vi "Get Altitude Data.vi"(8 "error in (no error)":errorcluster, 10 "Complete NMEA Sentences":string[](array[string]), 11 "VISA resource name":refnum<visa-resource-name>) -> (0 "error out":errorcluster, 1 "Altitude Data":cluster{"Timestamp":timestamp, "Altitude":dbl}[](array[cluster]), 2 "Complete NMEA Sentences (Copy)":string[](array[string]), 3 "VISA resource name out":refnum<visa-resource-name>)   [LabVIEW 2009]
doc: "Parses out the altitude data from all of the sentences that Read Raw.vi outputs, and passes through a complete copy of those sentences. Can be used in conjunction with other advanced \"Get\" VIs. See u-blox 5 Series Acquire and Chart GPS Advanced.vi for an example of how to use this VI.\n\nNote that the VISA Resource is not required, since this VI is a helper that does not actually interact with the device. The VISA Resource can be used, however, to clarify programming and maintain uniformity."
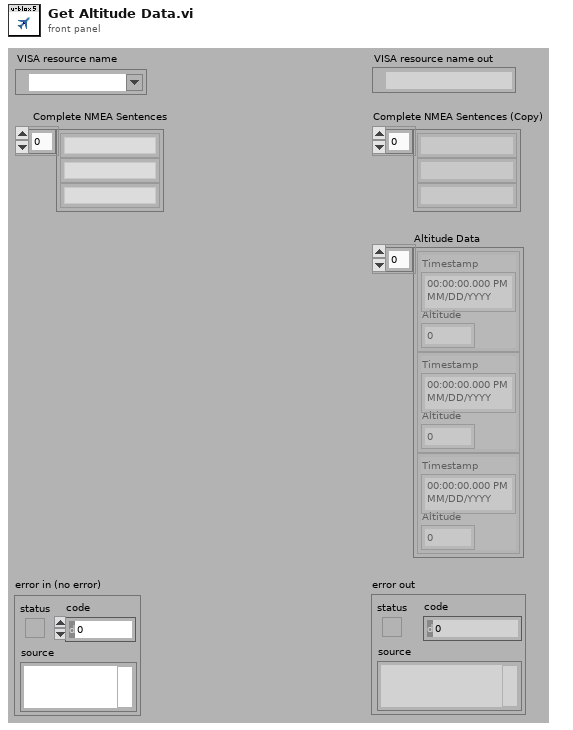
[diagram p1: front panel]
types:
  T1 = typedef "GGA Data.ctl" = cluster{"time of fix":cluster{"included?":bool, "time":timestamp}, "latitude":cluster{"included?":bool, "latitude (deg)":dbl}, "longitude":cluster{"included?":bool, "longitude (deg)":dbl}, "fix quality":cluster{"included?":bool, "quality":u16}, "number of satellites in view":cluster{"included?":bool, "number of satellites":i8}, "horizontal dilution of precision":cluster{"included?":bool, "horizontal DOP":dbl}, "altitude above mean sea level":cluster{"included?":bool, "altitude (m)":dbl}, "height of geoid above WGS84":cluster{"included?":bool, "height of geoid (m)":dbl}, "time since last DGPS update":cluster{"included?":bool, "time (s)":dbl}, "DGPS station ID number":cluster{"included?":bool, "station ID number":dbl}}
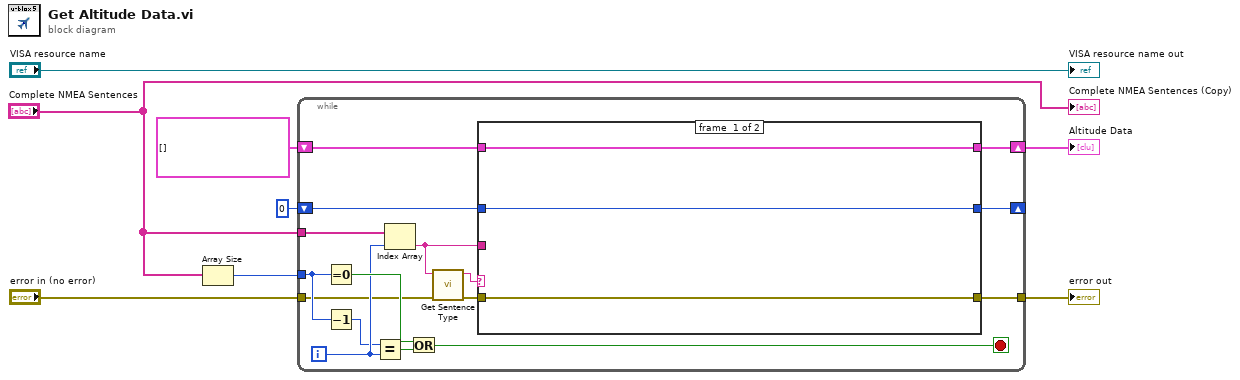
[diagram p0: block diagram]
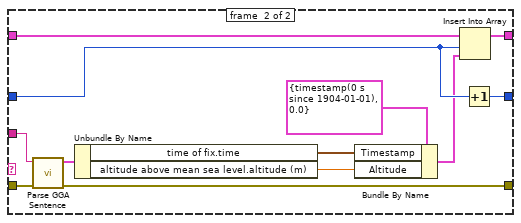
[diagram p2: hidden frame]
diagram:
  n1 = Array Size(array="Complete NMEA Sentences") -> (size(s)=w7:i32)
  n2 = while {
    tunnel: "Complete NMEA Sentences" -> [w24]
    shift-right: [w22] -> w1
    shift-left: cluster{"Timestamp":timestamp, "Altitude":dbl}[] [] -> [w21]
    tunnel: w7 -> [w18]
    tunnel: "error in (no error)" -> [w12]
    tunnel: [w23] -> w5
    shift-right: [w19] -> _
    shift-left: 0 -> [w20]
    i -> [w14]
    stop <- w16 stop-if-true
    n3 = Equal To 0?(x=w18) -> (x = 0?=w17:bool)
    n4 = Decrement(x=w18) -> (x-1=w13:i32)
    n5 = Equal?(x=w13, y=w14) -> (x = y?=w15:bool)
    n6 = Index Array(array=w24, index=w14) -> (element=w11:string)
    n7 = Or(x=w17, y=w15) -> (x .or. y?=w16:bool)
    n8 = call "Get Sentence Type.vi"("error in (no error)"=w12, "sentence"=w11) -> ("error out"=w9:errorcluster, "sentence type"=w10:string)  [unwired: 7 in, 1 out]
    n9 = case shown="\"GPGGA\"" w10 {
      tunnel: w11 -> [_ w29]
      tunnel: w9 -> [w27 w30]
      tunnel: [w27 w31] -> w23
      tunnel: [w26 w39] -> w22
      tunnel: w21 -> [w26 w38]
      tunnel: w20 -> [w25 w34]
      tunnel: [w25 w37] -> w19
      frame #0 {
      }
      frame #1 {
        n10 = call "Parse GGA Sentence.vi"("error in (no error)"=w30, "GGA sentence"=w29) -> ("error out"=w31:errorcluster, "GGA data"=w28:T1)  [unwired: 8 in]
        n11 = Unbundle By Name(w28) -> ("time of fix.time"=w32:timestamp, "altitude above mean sea level.altitude (m)"=w35:dbl)
        n12 = Bundle By Name(cluster=cluster{"Timestamp":timestamp, "Altitude":dbl} {"Timestamp"=timestamp(0 s since 1904-01-01), "Altitude"=0.0}, "Timestamp"=w32, "Altitude"=w35) -> (w33:cluster{"Timestamp":timestamp, "Altitude":dbl})
        n13 = Insert Into Array(array=w38, index=w34, new element=w33) -> (w39:cluster{"Timestamp":timestamp, "Altitude":dbl}[])
        n14 = Increment(x=w34) -> (x+1=w37:i32)
      }
    }
  }
  "error out" <- w5
  "Altitude Data" <- w1
  "VISA resource name out" <- "VISA resource name"
  "Complete NMEA Sentences (Copy)" <- "Complete NMEA Sentences"
